vi "myRIO_BRig_RT__Case_Exp_State_endTrial1.vi"(9 "input_spout":enum16{"Left", "Right"}(ring), 10 "input_dataBlock":u16[][](array[numeric]), 11 "input_dataCurrent":u16[](array[numeric])) -> (2 "output_dataBlock":u16[][](array[numeric]), 3 "output_dataCurrent":u16[](array[numeric]))   [LabVIEW 2014]
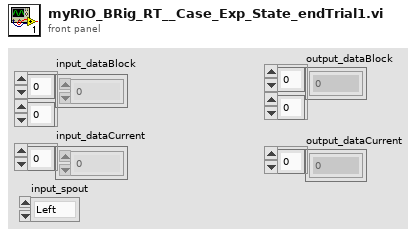
[diagram p1: front panel]
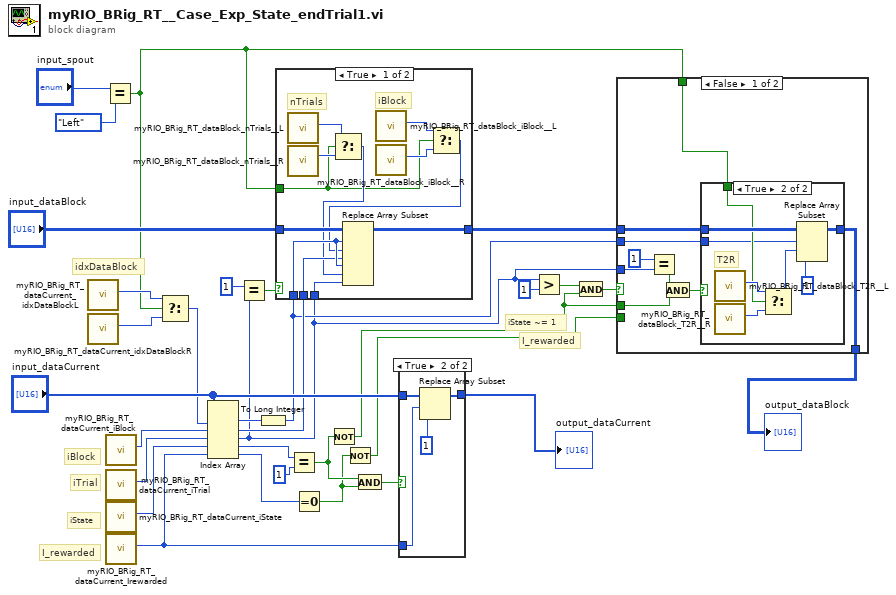
[diagram p0: block diagram]
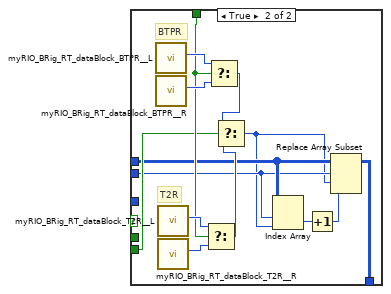
[diagram p3: hidden frame]
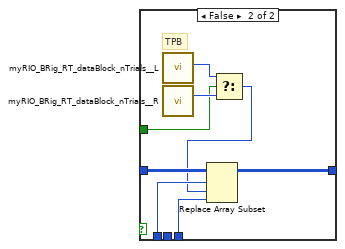
[diagram p4: hidden frame]
diagram:
  # "I_rewarded"
  # "iState ~= 1"
  # "iBlock"
  # "I_rewarded"
  # "iState"
  # "iTrial"
  # "idxDataBlock"
  n1 = call "myRIO_BRig_RT_dataCurrent_idxDataBlockL.vi"() -> ("output_idxDataBlock__L"=w31:i32)  [unwired: 11 in]
  n2 = call "myRIO_BRig_RT_dataCurrent_idxDataBlockR.vi"() -> ("output_idxDataBlock__R"=w32:i32)  [unwired: 11 in]
  n3 = Equal?(x="input_spout", y=enum16{"Left", "Right"}."Left") -> (x = y?=w4:bool)
  n4 = call "myRIO_BRig_RT_dataCurrent_iBlock.vi"() -> ("output_iBlock"=w19:i32)  [unwired: 11 in]
  n5 = call "myRIO_BRig_RT_dataCurrent_iTrial.vi"() -> ("output_iTrial"=w28:i32)  [unwired: 11 in]
  n6 = call "myRIO_BRig_RT_dataCurrent_iState.vi"() -> ("output_iState"=w27:i32)  [unwired: 11 in]
  n7 = call "myRIO_BRig_RT_dataCurrent_Irewarded.vi"() -> ("output_I_rewarded"=w23:i32)  [unwired: 11 in]
  n8 = Select(t=w31, s=w4, f=w32) -> (s? t:f=w16:i32)
  n9 = Index Array(array="input_dataCurrent", index #1=w16, index #2=w19, index #3=w28, index #4=w27, index #5=w23) -> (element #1=w15:u16, element #2=w18:u16, element #3=w2:u16, element #4=w12:u16, element #5=w11:u16)
  n10 = Equal?(x=u16 1 ("y"), y=w2) -> (x = y?=w20:bool)
  n11 = To Long Integer(number=w15) -> (32bit integer=w13:i32)
  n12 = case shown="True" w20 {
    tunnel: w13 -> [w37 w48]
    tunnel: w18 -> [w36 _]
    tunnel: "input_dataBlock" -> [w44 w52]
    tunnel: [w43 w51] -> w7
    tunnel: w4 -> [w33 w47]
    tunnel: w2 -> [w38 w45]
    frame True {
      # "nTrials"
      # "iBlock"
      n13 = call "myRIO_BRig_RT_dataBlock_nTrials__L.vi"() -> ("output_nTrials__L"=w39:i32)  [unwired: 11 in]
      n14 = call "myRIO_BRig_RT_dataBlock_nTrials__R.vi"() -> ("output_nTrials__R"=w40:i32)  [unwired: 11 in]
      n15 = Select(t=w39, s=w33, f=w40) -> (s? t:f=w34:i32)
      n16 = call "myRIO_BRig_RT_dataBlock_iBlock__L.vi"() -> ("output_iBlock__L"=w42:i32)  [unwired: 11 in]
      n17 = call "myRIO_BRig_RT_dataBlock_iBlock__R.vi"() -> ("output_iBlock__R"=w41:i32)  [unwired: 11 in]
      n18 = Select(t=w42, s=w33, f=w41) -> (s? t:f=w35:i32)
      n19 = Replace Array Subset(array=w44, new element #1=w36, index (row) #1=w37, index (col) #1=w35, new element #2=w38, index (row) #2=w37, index (col) #2=w34) -> (w43:u16[][])
    }
    frame False {
      # "TPB"
      n20 = call "myRIO_BRig_RT_dataBlock_nTrials__L.vi"() -> ("output_nTrials__L"=w49:i32)  [unwired: 11 in]
      n21 = call "myRIO_BRig_RT_dataBlock_nTrials__R.vi"() -> ("output_nTrials__R"=w50:i32)  [unwired: 11 in]
      n22 = Select(t=w49, s=w47, f=w50) -> (s? t:f=w46:i32)
      n23 = Replace Array Subset(array=w52, new element=w45, index (row)=w48, index (col)=w46) -> (w51:u16[][])
    }
  }
  n24 = Equal?(x=w12, y=u16 1) -> (x = y?=w10:bool)
  n25 = Equal To 0?(x=w11) -> (x = 0?=w9:bool)
  n26 = Not(x=w10) -> (.not. x?=w1:bool)
  n27 = Not(x=w9) -> (.not. x?=w8:bool)
  n28 = And(x=w10, y=w9) -> (x .and. y?=w25:bool)
  n29 = case shown="True" w25 {
    tunnel: "input_dataCurrent" -> [w53 w57]
    tunnel: w23 -> [_ w56]
    tunnel: [w53 w54] -> w22
    frame False {
    }
    frame True {
      n30 = Replace Array Subset(array=w57, new element=u16 1 ("new element/subarray"), index=w56) -> (w54:u16[])
    }
  }
  "output_dataCurrent" <- w22
  n31 = Greater?(x=w2, y=u16 1) -> (0:w6:bool)
  n32 = And(x=w6, y=w1) -> (x .and. y?=w5:bool)
  n33 = case shown="False" w5 {
    tunnel: w13 -> [w58 w80]
    tunnel: w8 -> [_ w84]
    tunnel: w7 -> [w61 w81]
    tunnel: w4 -> [w59 w85]
    tunnel: [w60 w76] -> w3
    tunnel: w2 -> [w66 _]
    tunnel: w1 -> [w63 _]
    frame False {
      n34 = Equal?(x=u16 1 ("y"), y=w66) -> (x = y?=w64:bool)
      n35 = And(x=w64, y=w63) -> (x .and. y?=w62:bool)
      n36 = case shown="True" w62 {
        tunnel: w61 -> [w67 w74]
        tunnel: [w67 w75] -> w60
        tunnel: w59 -> [_ w71]
        tunnel: w58 -> [_ w70]
        frame False {
        }
        frame True {
          # "T2R"
          n37 = call "myRIO_BRig_RT_dataBlock_T2R__L.vi"() -> ("output_T2R__L"=w72:i32)  [unwired: 11 in]
          n38 = call "myRIO_BRig_RT_dataBlock_T2R__R.vi"() -> ("output_T2R__R"=w73:i32)  [unwired: 11 in]
          n39 = Select(t=w72, s=w71, f=w73) -> (s? t:f=w69:i32)
          n40 = Replace Array Subset(array=w74, new element=u16 1 ("new element/subarray"), index (row)=w70, index (col)=w69) -> (w75:u16[][])
        }
      }
    }
    frame True {
      # "T2R"
      # "BTPR"
      n41 = call "myRIO_BRig_RT_dataBlock_BTPR__L.vi"() -> ("output_BTPR__L"=w88:i32)  [unwired: 11 in]
      n42 = call "myRIO_BRig_RT_dataBlock_BTPR__R.vi"() -> ("output_BTPR__R"=w89:i32)  [unwired: 11 in]
      n43 = call "myRIO_BRig_RT_dataBlock_T2R__L.vi"() -> ("output_T2R__L"=w86:i32)  [unwired: 11 in]
      n44 = call "myRIO_BRig_RT_dataBlock_T2R__R.vi"() -> ("output_T2R__R"=w87:i32)  [unwired: 11 in]
      n45 = Select(t=w86, s=w85, f=w87) -> (s? t:f=w82:i32)
      n46 = Select(t=w88, s=w85, f=w89) -> (s? t:f=w83:i32)
      n47 = Select(t=w83, s=w84, f=w82) -> (s? t:f=w79:i32)
      n48 = Index Array(array=w81, index (row)=w80, index (col)=w79) -> (element=w78:u16)
      n49 = Increment(x=w78) -> (x+1=w77:u16)
      n50 = Replace Array Subset(array=w81, new element=w77, index (row)=w80, index (col)=w79) -> (w76:u16[][])
    }
  }
  "output_dataBlock" <- w3
